vi "稱號-一色狂徒.vi"() -> ()   [LabVIEW 2014]
panel:
  in  "退出視窗":bool
  # "恭喜獲得稱號:"
  # "骰出一次一色的機率只有1296分之1 啊!\n你能骰出十次，可以說是被神所祝福的好運人啊!"
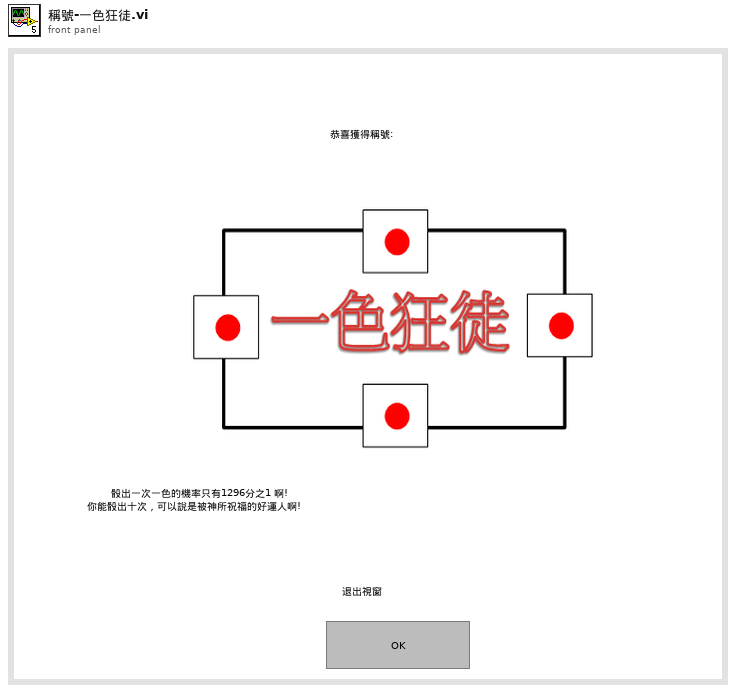
[diagram p1: front panel]
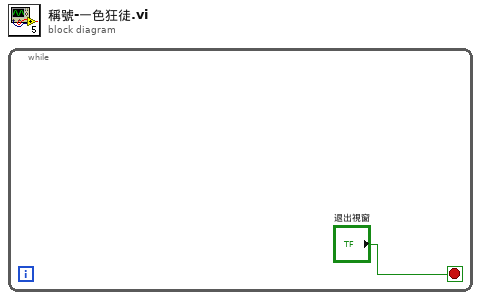
[diagram p0: block diagram]
diagram:
  n1 = while {
    stop <- "退出視窗" stop-if-true
  }
